vi "Parse configuration.vi"(8 "error in (no error)":errorcluster, 9 "Mode Name for Variant":string[](array[string]), 10 "Config File Sections":string[](array[string]), 11 "Refnum in":T1) -> (0 "error out":errorcluster, 3 "Variant array":variant[](array[variant]))   [LabVIEW 2020]
uses:
  <vilib>/Utility/config.llb/Config Data RefNum.ctl
  <vilib>/Utility/config.llb/Read Key (String).vi
  <vilib>/Utility/config.llb/NI_LVConfig.lvlib
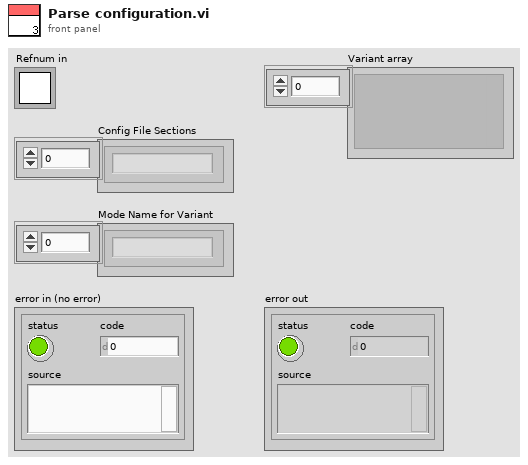
[diagram p1: front panel]
types:
  T1 = typedef "NI_LVConfig.lvlib/Config Data RefNum.ctl" = refnum<k1>
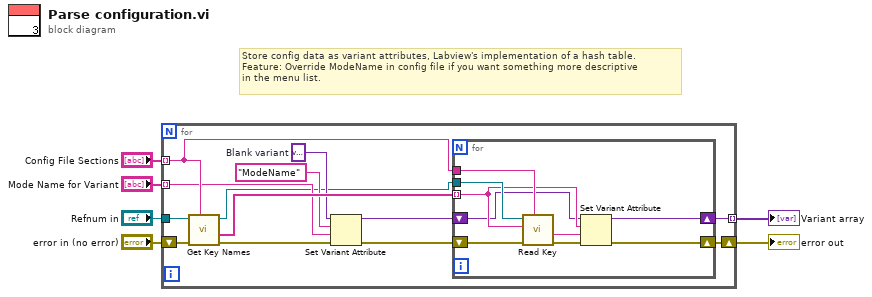
[diagram p0: block diagram]
diagram:
  # "Store config data as variant attributes, Labview's implementation of a hash table.\nFeature: Override ModeName in config file if you want something more descriptive\nin the menu list."
  n1 = for {
    shift-right: [w15] -> w6
    shift-left: "error in (no error)" -> [w19]
    tunnel: "Config File Sections" -> [w16] mode=indexing
    tunnel: "Refnum in" -> [w18]
    tunnel: "Mode Name for Variant" -> [w11] mode=indexing
    tunnel: [w14] -> w5 mode=indexing
    w12 = variant  # Blank variant
    n2 = call <vilib>:"Get Key Names.vi"("section"=w16, "error in (no error)"=w19, "refnum"=w18) -> ("error out"=w10:errorcluster, "key names"=w17:string[], "refnum out"=w9:T1)  [unwired: 5 in, 1 out]
    n3 = Set Variant Attribute(Variant=w12, name="ModeName", value=w11, error in=w10) -> (Variant out=w7:variant, error out=w8:errorcluster)  [unwired: 1 out]
    n4 = for {
      tunnel: w17 -> [w22] mode=indexing
      tunnel: w16 -> [w28]
      tunnel: w9 -> [w27]
      shift-right: [w24] -> w15
      shift-left: w8 -> [w26]
      shift-right: [w20] -> w14
      shift-left: w7 -> [w21]
      n5 = call-poly <vilib>:"Read Key.vi"("section"=w28, "error in (no error)"=w26, "key"=w22, "refnum"=w27) -> ("error out"=w25:errorcluster, "value"=w23:string)  [unwired: 4 in, 2 out]
      n6 = Set Variant Attribute(Variant=w21, name=w22, value=w23, error in=w25) -> (Variant out=w20:variant, error out=w24:errorcluster)  [unwired: 1 out]
    }
  }
  "error out" <- w6
  "Variant array" <- w5
